vi "GigE Vision Auto Packet Size.vi"(8 "error in (no error)":errorcluster, 11 "Camera in":refnum<class "Camera.lvclass">) -> (0 "error out":errorcluster, 2 "Packet Size":i32, 3 "Camera":refnum<class "Camera.lvclass">)   [LabVIEW 2020, in "Camera.lvclass"]
doc: "Automatically determine the biggest packet size that can be used data streaming, and set GevSCPSPacketSize value accordingly. This function relies on the GevSCPSFireTestPacket feature. If this feature is not available, the packet size will be set to a default value (1500 bytes)."
uses:
  Camera.lvclass
  Camera.lvclass/Camera.ctl
  bin/gindustrialcam_32-1.dll
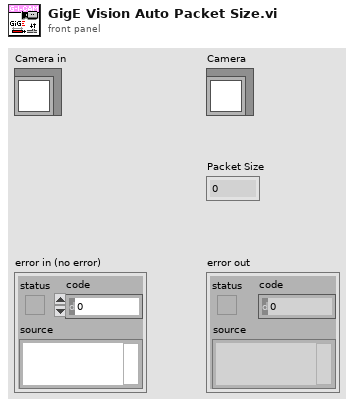
[diagram p1: front panel]
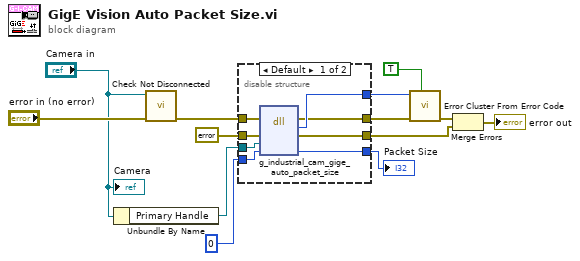
[diagram p0: block diagram]
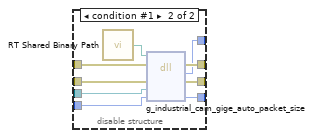
[diagram p2: hidden frame]
diagram:
  n1 = Unbundle By Name("Camera in") -> ("Primary Handle"=w3:refnum<data-value>)
  n2 = call "Check Not Disconnected.vi"("error in (no error)"="error in (no error)", "Camera in"="Camera in") -> ("error out"=w11:errorcluster)  [unwired: 9 in]
  n3 = disable-structure shown="Default" {
    disable-tunnel: w11 -> [w21 w30]
    disable-tunnel: errorcluster {"status"=FALSE, "code"=0, "source"=""} ("error constant") -> [w20 w25]
    disable-tunnel: [w19 w26] -> w8
    disable-tunnel: [w18 w27] -> w6
    disable-tunnel: [w17 w28] -> w5
    disable-tunnel: w3 -> [w16 w24]
    disable-tunnel: [w14 w22] -> w2
    disable-tunnel: 0 ("buffer size") -> [w15 w23]
    frame condition #0 (active) {
      n4 = dll-call lib="C:/serenial/lib/g-industrial-camera/LabVIEW/g_industrial_cam/bin/gindustrialcam_*-1.*" fn="g_industrial_cam_gige_auto_packet_size"(error in=w21, "err"=w20, "edvr"=w16, "size"=w15) -> (error out=w17:errorcluster, "Mg_Error"=w18:i32, "err"=w19:errorcluster, "size"=w14:i32)  [unwired: 3 in, 1 out]
    }
    frame condition #1 {
      n5 = call "RT Shared Binary Path.vi"() -> ("Path"=w29:path)
      n6 = dll-call lib="?" fn="g_industrial_cam_gige_auto_packet_size"(path in=w29, error in=w30, "err"=w25, "edvr"=w24, "size"=w23) -> (error out=w28:errorcluster, "Mg_Error"=w27:i32, "err"=w26:errorcluster, "size"=w22:i32)  [unwired: 2 in, 1 out]
    }
  }
  "Packet Size" <- w2
  n7 = call <vilib>:"Error Cluster From Error Code.vi"("show call chain? (False)"=TRUE, "error in (no error)"=w5, "error code (0)"=w6) -> ("error out"=w7:errorcluster)  [unwired: 6 in]
  n8 = Merge Errors(w7, w8) -> (→"error out":errorcluster)
  "Camera" <- "Camera in"
